vi "FPS Counter.vi"(8 "error in (no error)":errorcluster, 10 "Counter Reference":refnum<vi>, 11 "Phoenix in":refnum<class "Phoenix.lvclass">) -> (0 "error out":errorcluster, 2 "FPS":dbl, 3 "Phoenix out":refnum<class "Phoenix.lvclass">)   [LabVIEW 2022 SP3, in "Phoenix.lvlib" / "Phoenix.lvclass"]
uses:
  Phoenix.lvclass
  Phoenix.lvclass/Phoenix.ctl
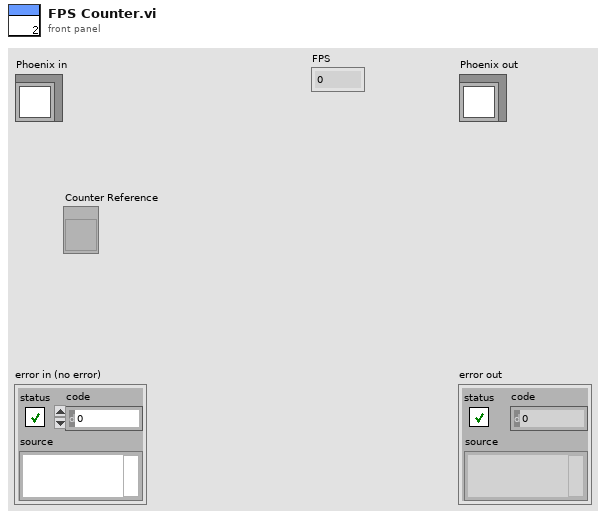
[diagram p1: front panel]
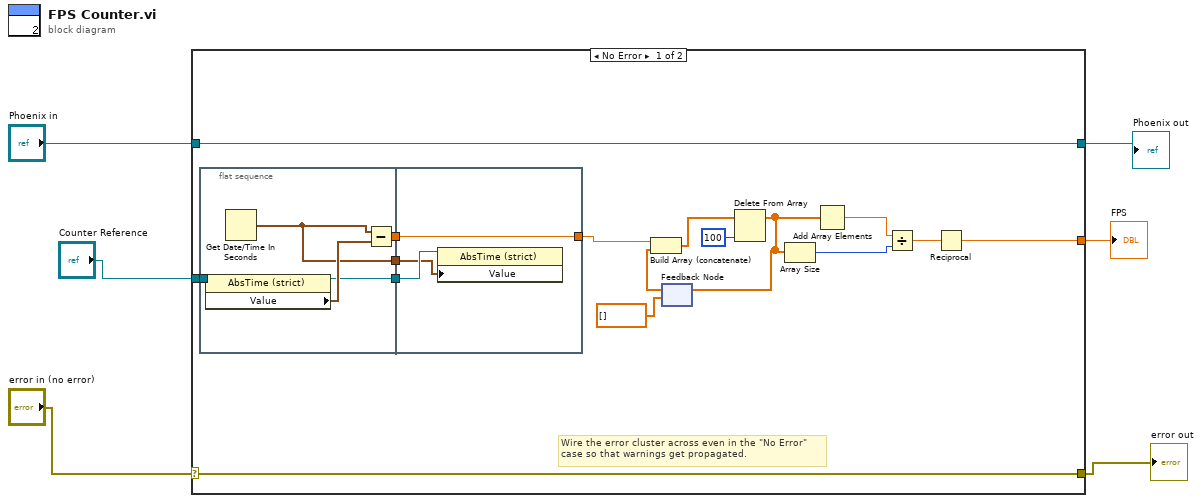
[diagram p0: block diagram]
diagram:
  n1 = case shown="No Error" "error in (no error)" {
    selector: "error in (no error)" -> [w22 w32]
    tunnel: [w22 w32] -> w3
    tunnel: [w12 _] -> w2
    tunnel: "Phoenix in" -> [w11 w31]
    tunnel: [w11 w31] -> w4
    tunnel: "Counter Reference" -> [w10 _]
    frame No Error {
      # "Wire the error cluster across even in the \"No Error\"\ncase so that warnings get propagated."
      n2 = flat-sequence {
        tunnel: w10 -> [w26]
        tunnel: [w27] -> w9
        tunnel: [w24] -> w8
        tunnel: [w23] -> w7
        tunnel: [w30] -> w13
        tunnel: w9 -> [w30]
        tunnel: w8 -> [w29]
        tunnel: w7 -> [w28]
        frame #0 {
          n3 = property class="AbsTime (strict)"(reference=w26) -> (reference out=w24:refnum<vi>, "Value"=w25:timestamp)  [unwired: 1 in, 1 out]
          n4 = Get Date/Time In Seconds() -> (seconds since 1Jan1904=w23:timestamp)
          n5 = Subtract(x=w23, y=w25) -> (x-y=w27:dbl)
        }
        frame #1 {
          n6 = property class="AbsTime (strict)"(reference=w29, "Value"=w28) -> ()  [unwired: 1 in, 2 out]
        }
      }
      n7 = feedback #1(dbl[] []) -> (w14:dbl[])
      n8 = Build Array (concatenate)(w13, w14) -> (w16:dbl[])
      n9 = Delete From Array(array=w16, index=100) -> (array with subset deleted=w20:dbl[])  [unwired: 1 in, 1 out]
      n10 = feedback-in #1(w20) -> ()
      n11 = Array Size(array=w20) -> (size(s)=w19:i32)
      n12 = Add Array Elements(numeric array=w20) -> (sum=w18:dbl)
      n13 = Divide(x=w18, y=w19) -> (x/y=w21:dbl)
      n14 = Reciprocal(x=w21) -> (1/x=w12:dbl)
    }
    frame Error {
    }
  }
  "error out" <- w3
  "Phoenix out" <- w4
  "FPS" <- w2
